vi "Configure Manifold.vi"(7 "Config Folder":path, 8 "error in (no error)":errorcluster, 11 "WorkTable Class in":refnum<class "WorkTable Class.lvclass">) -> (0 "error out":errorcluster, 3 "WorkTable Class out":refnum<class "WorkTable Class.lvclass">)   [LabVIEW 2011, in "WorkTable Class.lvclass"]
uses:
  WorkTable Class.lvclass
  <vilib>/Utility/config.llb/Read Key (U32).vi
  <vilib>/Utility/config.llb/Read Key (String).vi
  <vilib>/Utility/config.llb/NI_LVConfig.lvlib
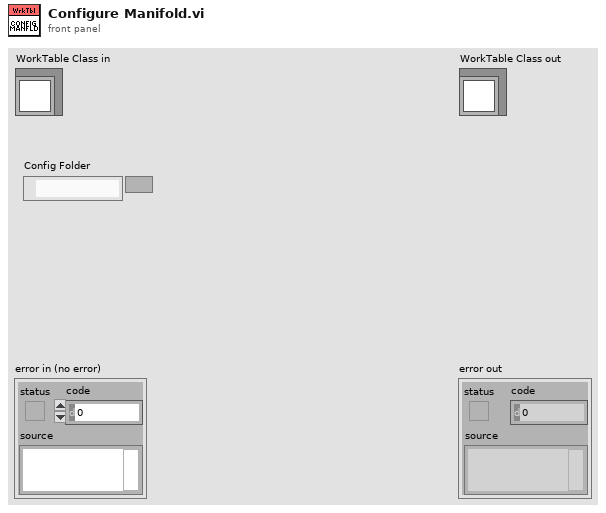
[diagram p1: front panel]
types:
  T1 = cluster{"Channels":cluster{"Enabled":bool, "Hardware Path":string}[]}
  T2 = typedef "NI_LVConfig.lvlib/Config Data RefNum.ctl" = refnum<k1>
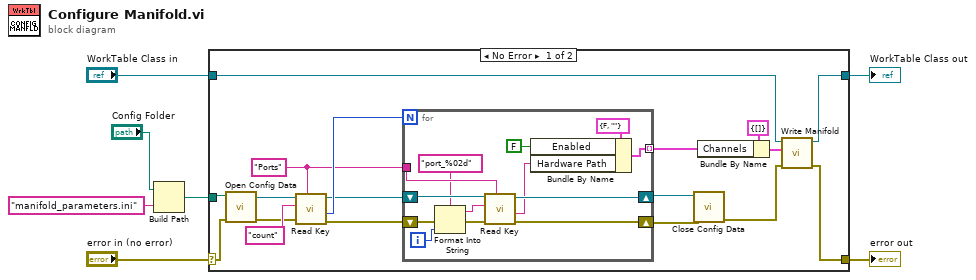
[diagram p0: block diagram]
diagram:
  n1 = Build Path(base path="Config Folder", name or relative path="manifold_parameters.ini") -> (appended path=w1:path)
  n2 = case shown="No Error" "error in (no error)" {
    selector: "error in (no error)" -> [w24 w40]
    tunnel: [w8 w40] -> w6
    tunnel: [w15 w39] -> w4
    tunnel: "WorkTable Class in" -> [w16 w39]
    tunnel: w1 -> [w25 _]
    frame No Error {
      w19 = "Ports" ("section")
      n3 = call <vilib>:"Open Config Data.vi"("error in (no error)"=w24, "configuration file path"=w25) -> ("error out"=w18:errorcluster, "refnum"=w23:T2)  [unwired: 7 in, 1 out]
      n4 = call-poly <vilib>:"Read Key.vi"("section"=w19, "error in (no error)"=w18, "key"="count", "refnum"=w23) -> ("error out"=w17:errorcluster, "value"=w21:u32, "refnum out"=w20:T2)  [unwired: 4 in, 1 out]
      n5 = for {
        N: w21 -> [_]
        tunnel: w19 -> [w38]
        shift-right: [w31] -> w11
        shift-left: w20 -> [w34]
        shift-right: [w30] -> w10
        shift-left: w17 -> [w36]
        tunnel: [w28] -> w12 mode=indexing
        i -> [w37]
        n6 = Format Into String(format string="port_%02d", error in=w36, w37) -> (resulting string=w33:string, error out=w35:errorcluster)  [unwired: 1 in]
        n7 = call-poly <vilib>:"Read Key.vi"("section"=w38, "error in (no error)"=w35, "key"=w33, "refnum"=w34) -> ("error out"=w30:errorcluster, "value"=w27:string, "refnum out"=w31:T2)  [unwired: 4 in, 1 out]
        n8 = Bundle By Name(cluster=cluster{"Enabled":bool, "Hardware Path":string} {"Enabled"=FALSE, "Hardware Path"=""} ("element"), "Enabled"=FALSE, "Hardware Path"=w27) -> (w28:cluster{"Enabled":bool, "Hardware Path":string})
      }
      n9 = call <vilib>:"Close Config Data.vi"("error in (no error)"=w10, "refnum"=w11) -> ("error out"=w9:errorcluster)  [unwired: 8 in, 1 out]
      n10 = Bundle By Name(cluster=T1 {"Channels"=[]} ("Manifold"), "Channels"=w12) -> (w13:T1)
      n11 = call-dynamic "Write Manifold.vi"("error in (no error)"=w9, "Manifold"=w13, "WorkTable Class in"=w16) -> ("error out"=w8:errorcluster, "WorkTable Class out"=w15:refnum<class "WorkTable Class.lvclass">)  [unwired: 7 in]
    }
    frame Error {
    }
  }
  "error out" <- w6
  "WorkTable Class out" <- w4
